vi "Add Run Sblock Creator.vi"(7 "SBlock type":string, 8 "Common Parameters":T1[](array[typedef]), 9 "Number of repetitions":u16, 10 "Script Path":path, 11 "FPGA Name":string) -> (0 "error out":errorcluster, 3 "Schedule Block out":refnum<class "Schedule Block.lvclass">)   [LabVIEW 2020, in "Scheduler.lvlib"]
uses:
  Scheduler.lvlib
  Run Utilities/Scan SBlock/Parameter name with value - GUI.ctl
  Run Utilities/Schedule Block/Schedule Block.lvclass
  Run Utilities/Scan SBlock/Scan SBlock.lvclass
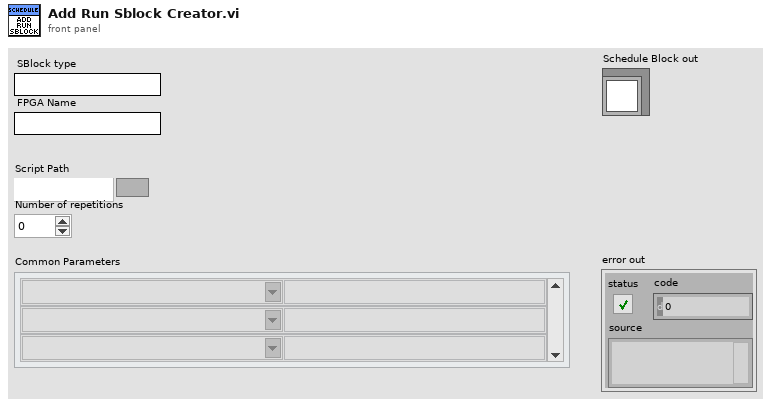
[diagram p1: front panel]
types:
  T1 = typedef "TALOS.lvlib/Run Utilities.lvlib/Scan SBlock.lvclass/Parameter name with value - GUI.ctl" = cluster{"Parameter Name":string, "Parameter Value":string}
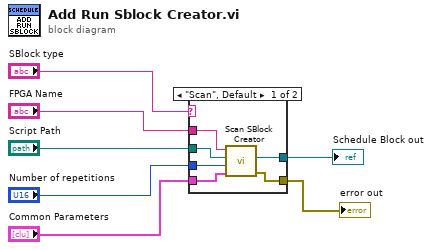
[diagram p0: block diagram]
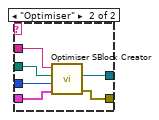
[diagram p2: hidden frame]
diagram:
  n1 = case shown="\"Scan\", Default" "SBlock type" {
    tunnel: "Number of repetitions" -> [w8 w16]
    tunnel: "Script Path" -> [w13 w17]
    tunnel: [w12 w18] -> w2
    tunnel: [w11 w19] -> w3
    tunnel: "FPGA Name" -> [w10 w14]
    tunnel: "Common Parameters" -> [w9 w15]
    frame "Scan", Default {
      n2 = call "Scan SBlock Creator.vi"("Common Parameters"=w9, "Number of repetitions"=w8, "Script Path"=w13, "FPGA Name"=w10) -> ("error out"=w12:errorcluster, "Schedule Block out"=w11:refnum<class "Schedule Block.lvclass">)  [unwired: 6 in]
    }
    frame "Optimiser" {
      n3 = call "Optimiser SBlock Creator.vi"("Common Parameters"=w15, "Number of repetitions"=w16, "Script Path"=w17, "FPGA Name"=w14) -> ("error out"=w18:errorcluster, "Schedule Block out"=w19:refnum<class "Schedule Block.lvclass">)  [unwired: 6 in]
    }
  }
  "Schedule Block out" <- w3
  "error out" <- w2
